vi "Add Node to Dictionary.vi"(8 "Error In":errorcluster, 9 "UID":string, 10 "New Node":refnum<class "Generic Node.lvclass">, 11 "Base Tree in":refnum<class "Base Tree.lvclass">) -> (3 "Base Tree out":refnum<class "Base Tree.lvclass">)   [LabVIEW 2017, in "Browser Core.lvlib" / "Base Tree.lvclass"]
doc: "Adds Node and UID to end of their respective arrays in the Node Dictionary."
uses:
  Base Tree.lvclass
  Node Classes/Generic Node/Generic Node.lvclass
  Base Tree.lvclass/Base Tree.ctl
panel:
  out "Error Out":errorcluster
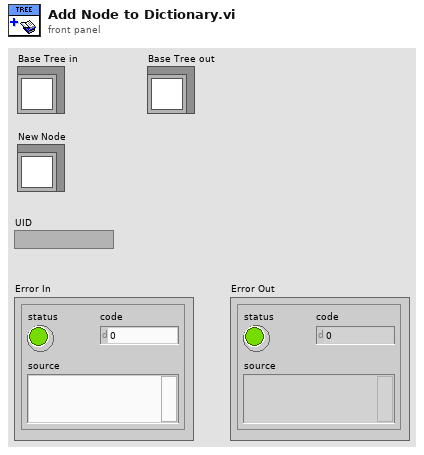
[diagram p1: front panel]
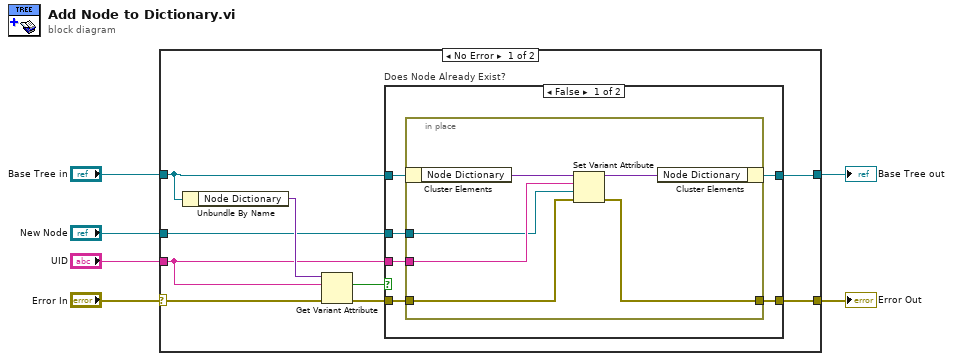
[diagram p0: block diagram]
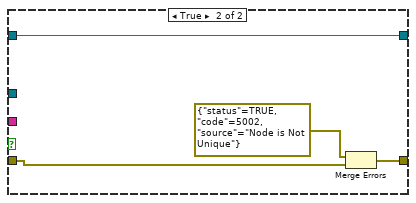
[diagram p2: hidden frame]
diagram:
  n1 = case shown="No Error" "Error In" {
    selector: "Error In" -> [w14 w32]
    tunnel: [w9 w33] -> w6
    tunnel: "UID" -> [w7 _]
    tunnel: "New Node" -> [w8 _]
    tunnel: "Base Tree in" -> [w10 w33]
    tunnel: [w11 w32] -> w1
    frame No Error {
      n2 = Unbundle By Name(w10) -> ("Node Dictionary"=w15:variant)
      n3 = Get Variant Attribute(Variant=w15, name=w7, error in=w14) -> (found=w12:bool, error out=w13:errorcluster)  [unwired: 1 in, 2 out]
      n4 = case "Does Node Already Exist?" shown="False" w12 {
        tunnel: w13 -> [w17 w30]
        tunnel: [w16 w31] -> w11
        tunnel: w10 -> [w21 w28]
        tunnel: [w20 w28] -> w9
        tunnel: w8 -> [w18 _]
        tunnel: w7 -> [w19 _]
        frame False {
          n5 = in-place {
            in-place-border: w19 -> [w26]
            in-place-border: w18 -> [w25]
            in-place-border: w17 -> [w23]
            in-place-border: [w22] -> w16
            n6 = in-place-cluster #1(w21) -> ("Node Dictionary"=w27:variant)
            n7 = Set Variant Attribute(Variant=w27, name=w26, value=w25, error in=w23) -> (Variant out=w24:variant, error out=w22:errorcluster)  [unwired: 1 out]
            n8 = in-place-cluster #1("Node Dictionary"=w24) -> (w20:refnum<class "Base Tree.lvclass">)
          }
        }
        frame True {
          n9 = Merge Errors(errorcluster {"status"=TRUE, "code"=5002, "source"="Node is Not Unique"} ("error IO"), w30) -> (w31:errorcluster)
        }
      }
    }
    frame Error {
      # "Do Not Edit Dictionary on Error In"
    }
  }
  "Base Tree out" <- w6
  "Error Out" <- w1
